vi "读取二进制文件.vi"() -> ()   [LabVIEW 2010]
panel:
  in  "计数":i32
  in  "偏移量（字节）（0）":i64
  out "读取的数据":dbl[][](graph)
  in  "停止":bool
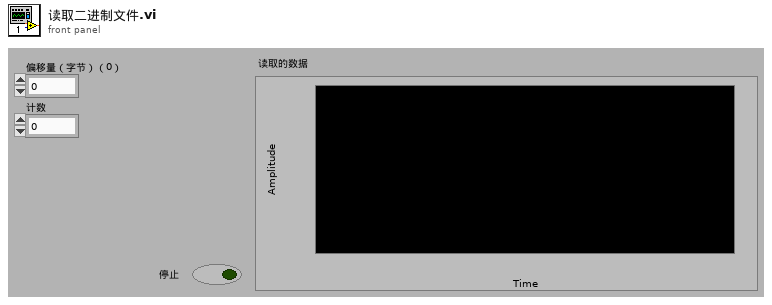
[diagram p1: front panel]
types:
  T1 = enum16{"big-endian, network order", "native, host order", "little-endian"}
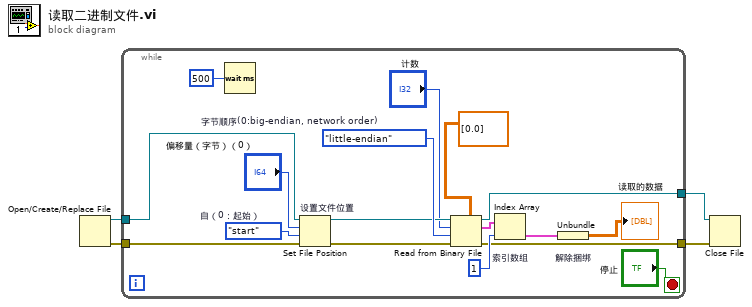
[diagram p0: block diagram]
diagram:
  n1 = Open/Create/Replace File() -> (refnum out=w4:refnum<file>, error out=w2:errorcluster)  [unwired: 6 in, 1 out]
  n2 = while {
    tunnel: w4 -> [w15]
    tunnel: [w13] -> w3
    tunnel: w2 -> [w9]
    tunnel: [w8] -> w1
    stop <- "停止" stop-if-true
    w12 = enum16{"start", "end", "current"}."start"  # 自（0：起始）
    w20 = T1."little-endian"  # 字节顺序(0:big-endian, network order)
    n3 = Wait (ms)(milliseconds to wait=u32 500 ("等待时间（毫秒）")) -> ()  [unwired: 1 out]
    n4 = Set File Position "设置文件位置"(offset (in bytes) (0)="偏移量（字节）（0）", refnum=w15, from (0:start)=w12, error in=w9) -> (refnum out=w14:refnum<file>, error out=w10:errorcluster)
    n5 = Read from Binary File(5:dbl[][] [[0.0]], 8:w10, 9:w20, 10:"计数", 11:w14) -> (0:w8:errorcluster, 2:w6:cluster{dbl[][]}[], 3:w13:refnum<file>)  [unwired: 1 in, 1 out]
    n6 = Index Array "索引数组"(array=w6, index=1 ("索引")) -> (element=w16:cluster{dbl[][]})
    n7 = Unbundle "解除捆绑"(w16) -> (→"读取的数据":dbl[][])
  }
  n8 = Close File(refnum=w3, error in=w1) -> ()  [unwired: 2 out]
